vi "Setup Connection.vi"(0 "Cal Standard Sim in":refnum<class "Cal Standard Sim.lvclass">, 5 "Path Name":string, 11 "error in (no error)":errorcluster) -> (4 "Cal Standard Sim out":refnum<class "Cal Standard Sim.lvclass">, 15 "error out":errorcluster)   [LabVIEW 2023, in "RFFixtureCharact.Instruments.lvlib" / "Cal Standard Sim.lvclass"]
uses:
  Cal Standard Sim.lvclass
  C:/srd-semi-rfcal-software/AuxTools/STSRFFixtureCharactUtility/Source/Code Modules/Fixture/Instruments/Cal Standard/Cal Standard Base/Cal Standard Base.lvclass
  Cal Standard Base/Cal Standard Base.lvclass/Cal Standard Base.ctl
  Cal Standard Base/Properties/Read Path Connection Map.vi
  Cal Standard Base/Properties/Read Instrument Info.vi
  Cal Standard Base/Properties/Write Path Connection Map.vi
  <vilib>/Utility/error.llb/Trim Whitespace One-Sided.vi
  Common/RFCalAndFixtureCharact.Common.lvlib
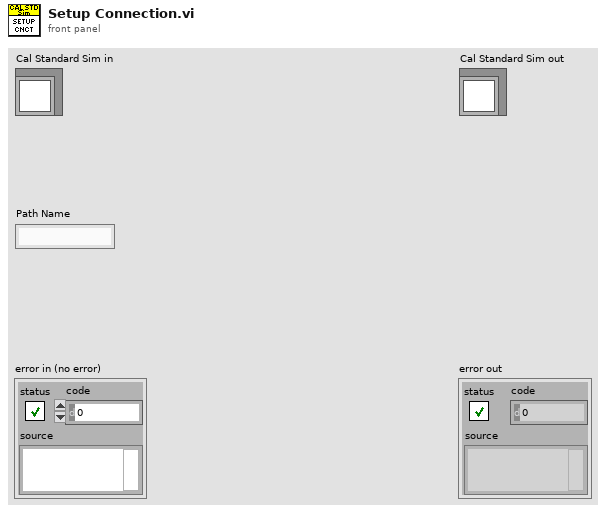
[diagram p1: front panel]
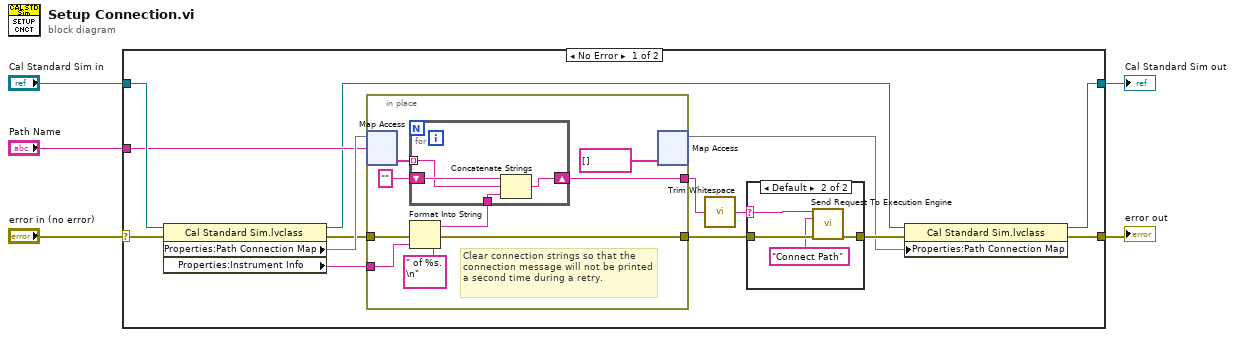
[diagram p0: block diagram]
diagram:
  n1 = case shown="No Error" "error in (no error)" {
    selector: "error in (no error)" -> [w19 w39]
    tunnel: [w14 w39] -> w2
    tunnel: [w11 w38] -> w1
    tunnel: "Cal Standard Sim in" -> [w18 w38]
    tunnel: "Path Name" -> [w16 _]
    frame No Error {
      n2 = property class="Cal Standard Sim.lvclass"(reference=w18, error in=w19) -> (reference out=w12:refnum<class "Cal Standard Sim.lvclass">, error out=w7:errorcluster, "Properties:Path Connection Map"=w17:map{string, string[]}, "Properties:Instrument Info"=w8:string)
      n3 = in-place {
        in-place-border: [w27] -> w10
        in-place-border: w8 -> [w24]
        in-place-border: w7 -> [w23]
        in-place-border: [w21] -> w6
        # "Clear connection strings so that the connection message will not be printed a second time during a retry."
        n4 = in-place-map #1(w17, w16) -> (w26:string[])  [unwired: 1 in, 1 out]
        n5 = Format Into String(format string=" of %s.\n" ("message"), error in=w23, w24) -> (resulting string=w20:string, error out=w21:errorcluster)  [unwired: 1 in]
        n6 = for {
          tunnel: w26 -> [w31] mode=indexing
          shift-right: [w30] -> w27
          shift-left: "" -> [w32]
          tunnel: w20 -> [w29]
          n7 = Concatenate Strings(w32, w31, w29) -> (w30:string)
        }
        n8 = in-place-map #1(string[] [] ("value")) -> (w13:map{string, string[]})  [unwired: 1 in, 2 out]
      }
      n9 = call <vilib>:"Trim Whitespace.vi"("string"=w10) -> ("trimmed string"=w9:string)  [unwired: 1 in]
      n10 = case shown="Default" w9 {
        selector: w9 -> [_ w34]
        tunnel: w6 -> [w33 w37]
        tunnel: [w33 w35] -> w15
        frame "" {
        }
        frame Default {
          n11 = call "Send Request To Execution Engine.vi"("Request Message"=w34, "Request Header"="Connect Path", "error in (no error)"=w37) -> ("error out"=w35:errorcluster)  [unwired: 11 in, 1 out]
        }
      }
      n12 = property class="Cal Standard Sim.lvclass"(reference=w12, error in=w15, "Properties:Path Connection Map"=w13) -> (reference out=w11:refnum<class "Cal Standard Sim.lvclass">, error out=w14:errorcluster)
    }
    frame Error {
    }
  }
  "error out" <- w2
  "Cal Standard Sim out" <- w1
